vi "serail_test.vi"() -> ()   [LabVIEW 2016]
uses:
  <vilib>/Instr/_visa.llb/VISA Configure Serial Port (Instr).vi
panel:
  out "Okunan":string
  out "Yazılan":string
  out "x/y":dbl
  in  "Teta Aralık":dbl=10.0
  out "i":i32
  in  "Numeric Control":i32=360
  in  "Motor Driver Port":refnum<visa-resource-name>="COM3"
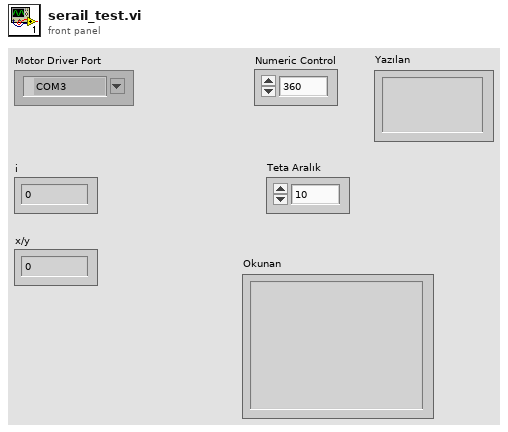
[diagram p1: front panel]
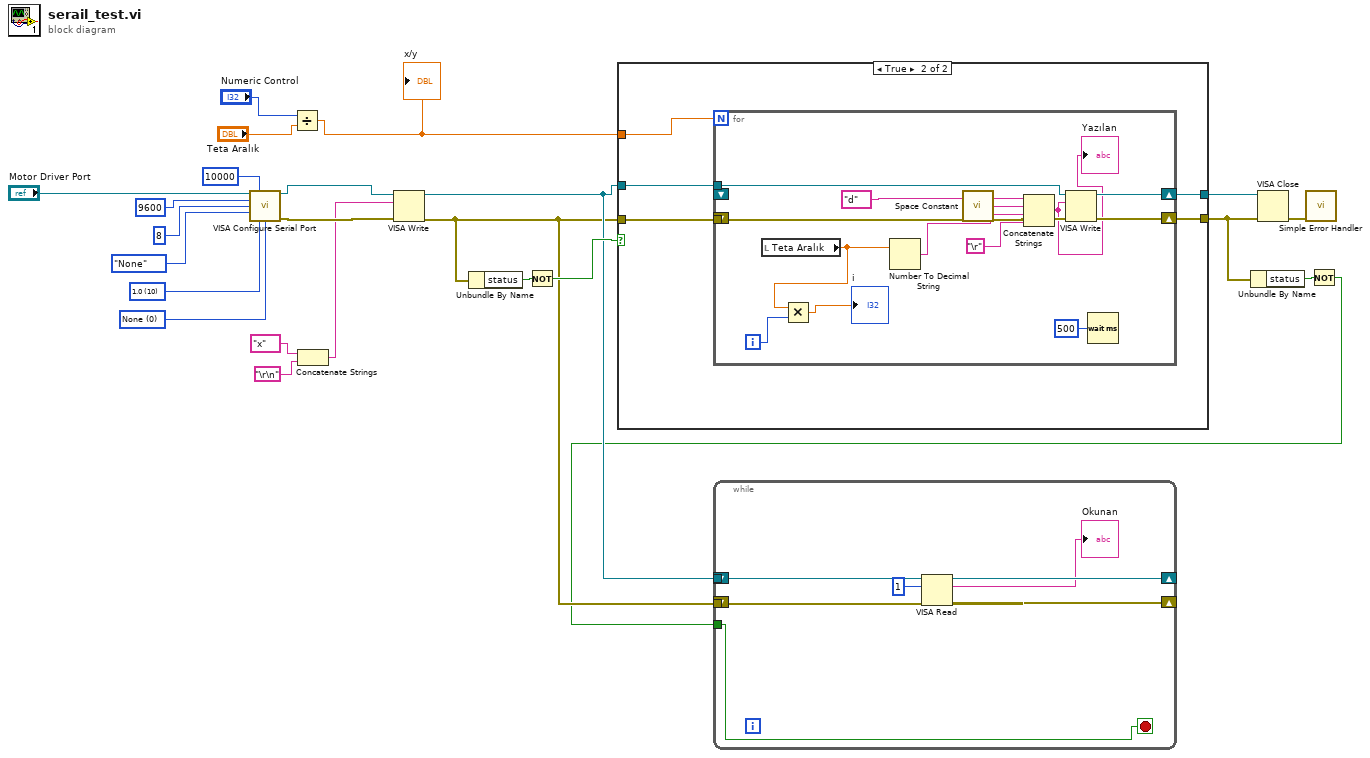
[diagram p0: block diagram]
diagram:
  w18 = u16 0 items=["None", "XON/XOFF", "RTS/CTS", "XON/XOFF & RTS/CTS", "DTR/DSR", "XON/XOFF & DTR/DSR"] ("flow control (0:none)")
  w19 = u16 10 items=["1.0"=10, "1.5"=15, "2.0"=20] ("stop bits (10: 1 bit)")
  n1 = call-poly "VISA Configure Serial Port"("VISA resource name"="Motor Driver Port", "timeout (10sec)"=u32 10000, "baud rate (9600)"=u32 9600, "data bits (8)"=u16 8, "parity (0:none)"=enum16{"None", "Odd", "Even", "Mark", "Space"}."None", "stop bits (10: 1 bit)"=w19, "flow control (0:none)"=w18) -> ("VISA resource name out"=w12:refnum<visa-resource-name>, "error out"=w11:errorcluster)  [unwired: 7 in]
  n2 = Divide(x="Numeric Control", y="Teta Aralık") -> (x/y=w13:dbl)
  "x/y" <- w13
  n3 = Concatenate Strings("x" ("string"), "\r\n") -> (w10:string)
  n4 = VISA Write(VISA resource name=w12, write buffer=w10, error in (no error)=w11) -> (VISA resource name out=w5:refnum<visa-resource-name>, error out=w2:errorcluster)  [unwired: 1 out]
  n5 = Unbundle By Name(w2) -> ("status"=w7:bool)
  n6 = Not(x=w7) -> (.not. x?=w6:bool)
  n7 = case shown="True" w6 {
    tunnel: [_ w29] -> w16
    tunnel: [_ w28] -> w3
    tunnel: w13 -> [_ w27]
    tunnel: w5 -> [_ w26]
    tunnel: w2 -> [_ w25]
    frame False {
    }
    frame True {
      n8 = for {
        N: w27 -> [_]
        tunnel: w26 -> [w41]
        tunnel: w25 -> [w40]
        shift-right: [w38] -> w29
        shift-left: _ -> [_]
        shift-right: [w39] -> w28
        shift-left: _ -> [_]
        i -> [w33]
        n9 = local read "Teta Aralık"() -> (w34:dbl)
        n10 = Multiply(x=w34, y=w33) -> (x*y=→"i":dbl)
        n11 = Number To Decimal String(number=w34) -> (decimal integer string=w35:string)  [unwired: 1 in]
        n12 = call <vilib>:"Space Constant.vi"() -> ("String"=w37:string)
        n13 = Concatenate Strings("d" ("string"), w37, w35, "\r") -> (w31:string)
        "Yazılan" <- w31
        n14 = VISA Write(VISA resource name=w41, write buffer=w31, error in (no error)=w40) -> (VISA resource name out=w38:refnum<visa-resource-name>, error out=w39:errorcluster)  [unwired: 1 out]
        n15 = Wait (ms)(milliseconds to wait=u32 500) -> ()  [unwired: 1 out]
      }
    }
  }
  n16 = Unbundle By Name(w3) -> ("status"=w4:bool)
  n17 = VISA Close(VISA resource name=w16, error in (no error)=w3) -> (error out=w17:errorcluster)
  n18 = call <vilib>:"Simple Error Handler.vi"("error in (no error)"=w17) -> ()  [unwired: 4 in, 5 out]
  n19 = Not(x=w4) -> (.not. x?=w1:bool)
  n20 = while {
    tunnel: w5 -> [w49]
    tunnel: w2 -> [w48]
    shift-right: [w46] -> _
    shift-left: _ -> [_]
    shift-right: [w47] -> _
    shift-left: _ -> [_]
    tunnel: w1 -> [w45]
    stop <- w45 stop-if-true
    n21 = VISA Read(VISA resource name=w49, byte count=u32 1, error in (no error)=w48) -> (VISA resource name out=w46:refnum<visa-resource-name>, read buffer=→"Okunan":string, error out=w47:errorcluster)  [unwired: 1 out]
  }
